vi "GetCCDPerformanceInfo.vi"(2 "Color":string, 3 "RO Speed Mode":dbl) -> (0 "Read Noise":dbl, 1 "Gain":dbl)   [LabVIEW 2015]
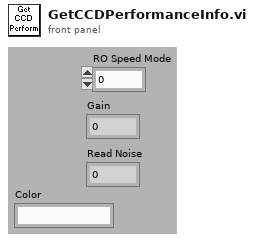
[diagram p1: front panel]
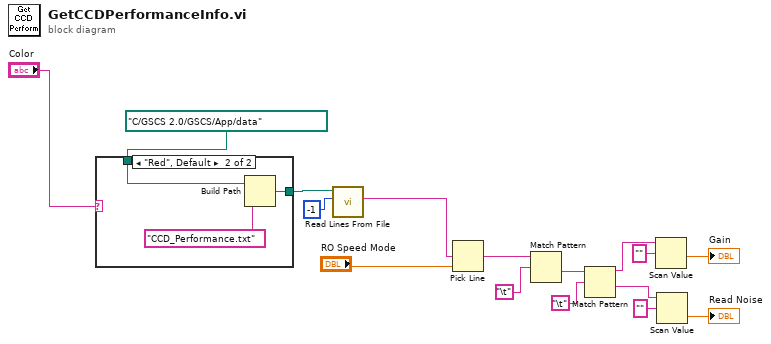
[diagram p0: block diagram]
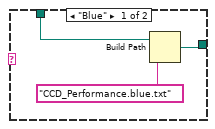
[diagram p2: hidden frame]
diagram:
  n1 = case shown="\"Red\", Default" "Color" {
    tunnel: [w17 w21] -> w3
    tunnel: path "C:/GSCS 2.0/GSCS/App/data" -> [w18 w20]
    frame "Blue" {
      n2 = Build Path(base path=w18, name or relative path="CCD_Performance.blue.txt" ("string")) -> (appended path=w17:path)
    }
    frame "Red", Default {
      n3 = Build Path(base path=w20, name or relative path="CCD_Performance.txt" ("string")) -> (appended path=w21:path)
    }
  }
  n4 = call <vilib>:"Read Lines From File.vi"("file path (dialog if empty)"=w3, "number of lines (all:-1)"=-1) -> ("line string"=w5:string)  [unwired: 4 in, 3 out]
  n5 = Pick Line(multi-line string=w5, line index="RO Speed Mode") -> (output string=w6:string)  [unwired: 1 in]
  n6 = Match Pattern(string=w6, regular expression="\t") -> (after substring=w15:string)  [unwired: 1 in, 3 out]
  n7 = Match Pattern(string=w15, regular expression="\t") -> (before substring=w9:string, after substring=w12:string)  [unwired: 1 in, 2 out]
  n8 = Scan Value(string=w9, format string="") -> (value=→"Gain":dbl)  [unwired: 1 in, 1 out]
  n9 = Scan Value(string=w12, format string="") -> (value=→"Read Noise":dbl)  [unwired: 1 in, 1 out]
